vi "SubVI_ReCluster_001.vi"(1 "Array":T1(array[cluster])) -> (0 "output cluster":cluster{string[], "Dissimilarity":dbl[][]})   [LabVIEW 2018]
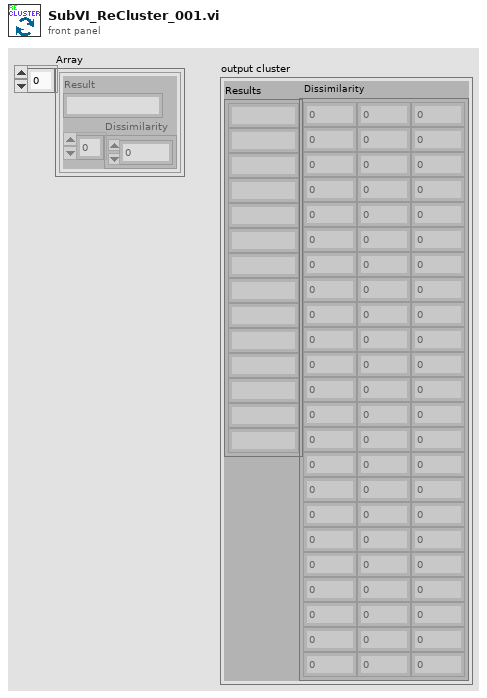
[diagram p1: front panel]
types:
  T1 = cluster{"Result":string, "Dissimilarity":dbl[]}[]
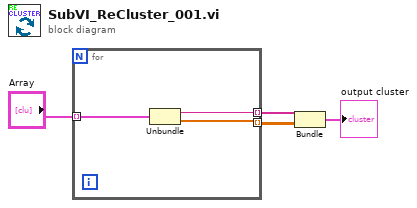
[diagram p0: block diagram]
diagram:
  n1 = for {
    tunnel: "Array" -> [w7] mode=indexing
    tunnel: [w6] -> w3 mode=indexing
    tunnel: [w5] -> w2 mode=indexing
    n2 = Unbundle(w7) -> ("Result"=w6:string, "Dissimilarity"=w5:dbl[])
  }
  n3 = Bundle(w3, "Dissimilarity"=w2) -> (→"output cluster":cluster{string[], "Dissimilarity":dbl[][]})  [unwired: 1 in]
